vi "Stop Trigger.vi"   [LabVIEW 2017, in "Sefram DAS220.lvlib"]
doc: "Stop recording on condition."
uses:
  <instrlib>/Sefram DAS220/Sefram DAS220.lvlib
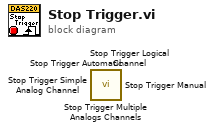
[diagram p0: block diagram]
diagram:
  n1 = call <instrlib>:"Stop Trigger Multiple Analogs Channels.vi"() -> ()  [unwired: 10 in, 2 out]
  n2 = call <instrlib>:"Stop Trigger Logical Channel.vi"() -> ()  [unwired: 10 in, 2 out]
  n3 = call <instrlib>:"Stop Trigger Simple Analog Channel.vi"() -> ()  [unwired: 10 in, 2 out]
  n4 = call <instrlib>:"Stop Trigger Manual.vi"() -> ()  [unwired: 10 in, 2 out]
  n5 = call <instrlib>:"Stop Trigger Automatic.vi"() -> ()  [unwired: 10 in, 2 out]
